vi "Write Current Set.vi"(0 "configuration file path":path, 1 "Current Set":u8[][](array[numeric]), 3 "error in (no error)":errorcluster) -> (7 "file path":path, 10 "error out":errorcluster)   [LabVIEW 2023]
uses:
  <vilib>/Utility/config.llb/Write Key (String).vi
  <vilib>/Utility/config.llb/NI_LVConfig.lvlib
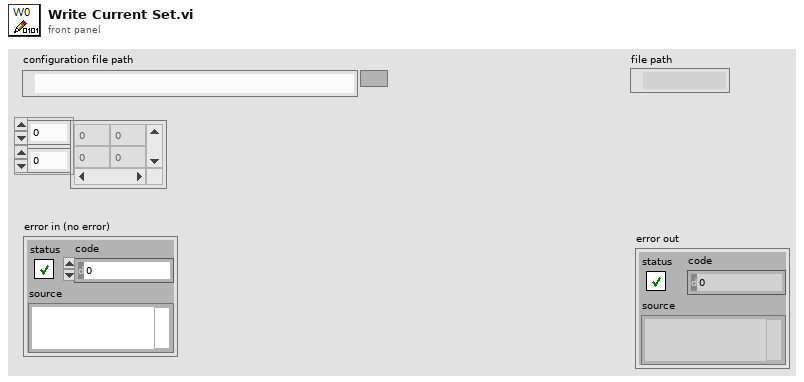
[diagram p1: front panel]
types:
  T1 = typedef "NI_LVConfig.lvlib/Config Data RefNum.ctl" = refnum<k1>
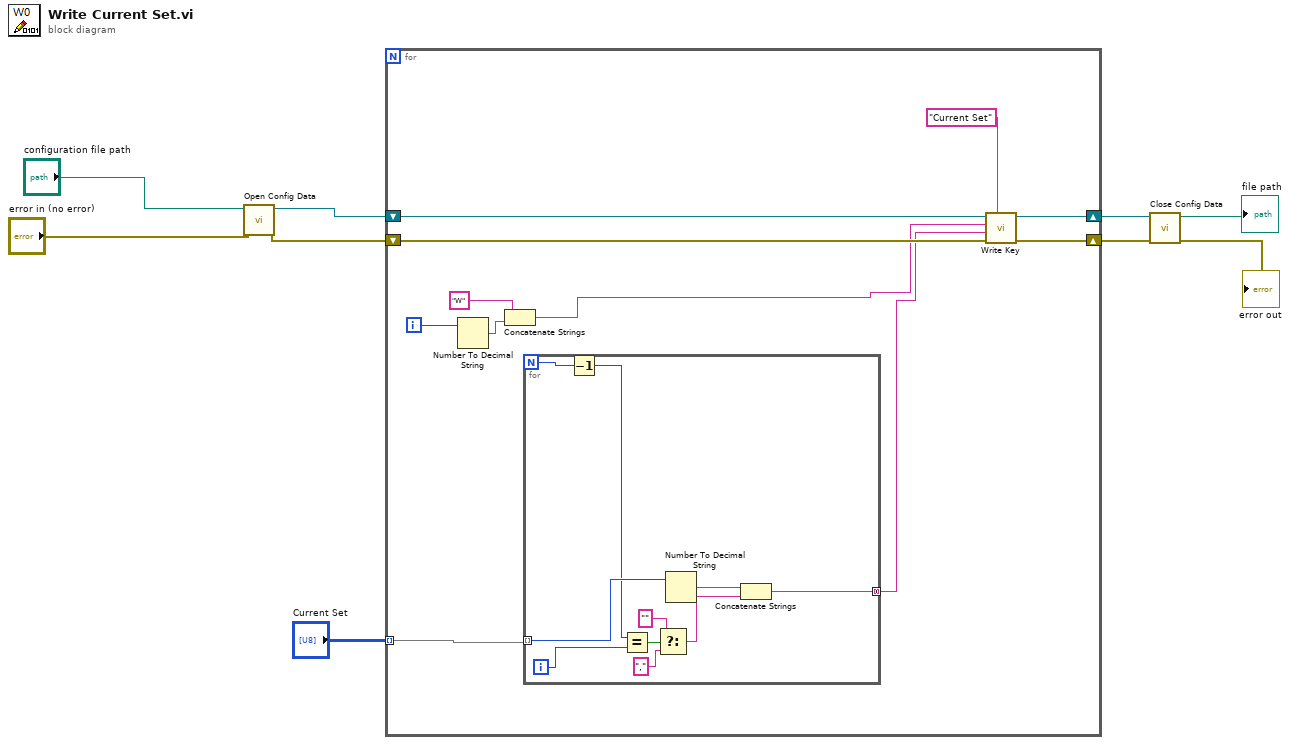
[diagram p0: block diagram]
diagram:
  n1 = call <vilib>:"Open Config Data.vi"("error in (no error)"="error in (no error)", "configuration file path"="configuration file path") -> ("error out"=w2:errorcluster, "refnum"=w3:T1)  [unwired: 7 in, 1 out]
  n2 = for {
    shift-right: [w18] -> w4
    shift-left: w3 -> [w17]
    shift-right: [w19] -> w5
    shift-left: w2 -> [w16]
    tunnel: "Current Set" -> [w10] mode=indexing
    i -> [w14]
    n3 = Number To Decimal String(number=w14) -> (decimal integer string=w13:string)  [unwired: 1 in]
    n4 = Concatenate Strings("W" ("string"), w13) -> (w11:string)
    n5 = for {
      N -> [w25]
      tunnel: w10 -> [w30] mode=indexing
      tunnel: [w28] -> w15 mode=concatenating
      i -> [w26]
      n6 = Decrement(x=w25) -> (x-1=w24:i32)
      n7 = Equal?(x=w24, y=w26) -> (x = y?=w27:bool)
      n8 = Select(t="", s=w27, f="," ("string")) -> (s? t:f=w23:string)
      n9 = Number To Decimal String(number=w30) -> (decimal integer string=w29:string)  [unwired: 1 in]
      n10 = Concatenate Strings(w29, w23) -> (w28:string)
    }
    n11 = call-poly <vilib>:"Write Key.vi"("section"="Current Set", "error in (no error)"=w16, "value"=w15, "key"=w11, "refnum"=w17) -> ("error out"=w19:errorcluster, "refnum out"=w18:T1)  [unwired: 4 in, 1 out]
  }
  n12 = call <vilib>:"Close Config Data.vi"("error in (no error)"=w5, "refnum"=w4) -> ("error out"=→"error out":errorcluster, "file path"=→"file path":path)  [unwired: 8 in]
